vi "SynchIO.USB4431.DVRtoRef.vi"(10 "Ref":T1) -> (2 "Ref":u32 format="%08x")   [LabVIEW 2016, in "SynchIO.PXI-4461.lvclass"]
doc: "JKI State Machine Objects (SMO) 1.0.0.5\nJKI - JKI\nCopyright (c) 2016, JKI"
uses:
  SynchIO.PXI-4461.lvclass
  Typedefs/PrivateData--Ref.ctl
  Typedefs/PrivateData--Cluster.ctl
  Typedefs/Configuration--Cluster.ctl
  Typedefs/PublicEvents--Cluster.ctl
  Typedefs/DataChanged--EventData--Cluster.ctl
  Typedefs/PublicEvents--SynchIO.USB4431.Initialize.ctl
  Typedefs/ProtectedEvents--Cluster.ctl
  Typedefs/API Inputs--Cluster.ctl
  Typedefs/PrivateEvents--Cluster.ctl
  Typedefs/PrivateEvents--SynchIO.USB4431.Initialize.ctl
  Typedefs/PrivateEvents--SynchIO.USB4431.Init.ctl
  Typedefs/PrivateEvents--SynchIO.USB4431.Init-Event.ctl
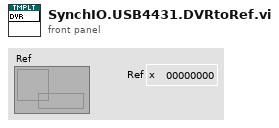
[diagram p1: front panel]
types:
  T1 = typedef "SynchIO.PXI-4461.lvclass/PrivateData--Ref.ctl" = refnum<data-value>
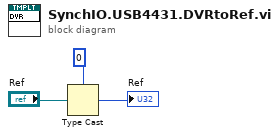
[diagram p0: block diagram]
diagram:
  n1 = Type Cast(type=u32 0 ("Ref"), x="Ref") -> (*(type *) &x=→"Ref":u32)
